vi "MT Measure QAM Quadrature Impairments.vi"(0 "recovered complex waveform":T6={"t0"=0.0, "dt"=1.0, "Y"=[]} {"Y" format="%.3f"; "dt" format="%^.2e"; "t0" format="%.4f"}, 1 "QAM system parameters":T3={"samples per symbol (16)"=16, "symbol map"=[]} {"symbol map" format="%.3f"}, 5 "input bit stream":i8[](array[numeric]), 7 "impairment measurement window":T4={"start index (symbols)"=0, "width (symbols) (-1: all)"=-1}, 9 "EVM normalization type":enum16{"Peak ", "RMS "}(ring), 11 "error in (no error)":errorcluster, 12 "impairment definition":enum16{"Vertical Shear", "Axis Shear"}(ring), 13 "reset? (T)":bool=TRUE) -> (2 "magnitude error":T1 {"individual symbol measurements (%)" format="%.2f"; "peak measurement (%)" format="%.2f"; "RMS measurement (%)" format="%.2f"}, 3 "DC offset measurements":T5 {"origin offset (dB)" format="%.2f"; "Q (%)" format="%.2f"; "I (%)" format="%.2f"}, 4 "IQ gain imbalance (dB)":dbl format="%.2f", 6 "phase error":T2 {"individual symbol measurements (deg)" format="%.2f"; "peak measurement (deg)" format="%.2f"; "RMS measurement (deg)" format="%.2f"}, 8 "EVM":T1 {"individual symbol measurements (%)" format="%.2f"; "peak measurement (%)" format="%.2f"; "RMS measurement (%)" format="%.2f"}, 10 "modulation error ratio (dB)":dbl format="%.2f", 14 "quadrature skew (deg)":dbl format="%.2f", 15 "error out":errorcluster)   [LabVIEW 2020, in "niDMT.lvlib"]
doc: "This polymorphic instance calculates and reports quadrature-amplitude modulation (QAM) quadrature impairments."
uses:
  <vilib>/addons/Modulation/niDMT.lvlib
  <vilib>/addons/Modulation/Analog/controls/Complex Data Waveform.ctl
  <vilib>/addons/Modulation/niAMT.lvlib
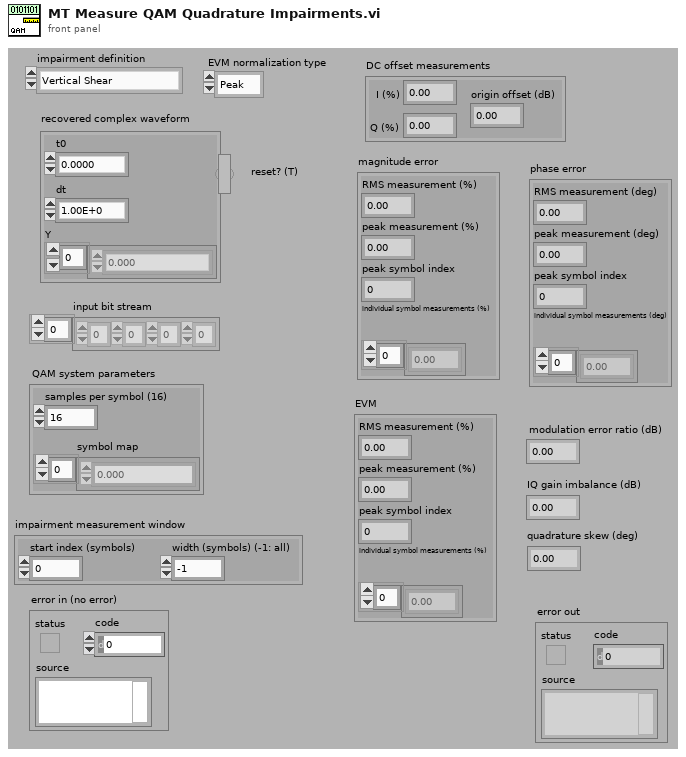
[diagram p1: front panel]
types:
  T1 = cluster{"RMS measurement (%)":dbl, "peak measurement (%)":dbl, "peak symbol index":i32, "individual symbol measurements (%)":dbl[]}
  T2 = cluster{"RMS measurement (deg)":dbl, "peak measurement (deg)":dbl, "peak symbol index":i32, "individual symbol measurements (deg)":dbl[]}
  T3 = cluster{"samples per symbol (16)":i32, "symbol map":cdb[]}
  T4 = cluster{"start index (symbols)":i32, "width (symbols) (-1: all)":i32}
  T5 = cluster{"I (%)":dbl, "Q (%)":dbl, "origin offset (dB)":dbl}
  T6 = typedef "niAMT.lvlib/Complex Data Waveform.ctl" = cluster{"t0":dbl, "dt":dbl, "Y":cdb[]}
  T7 = enum16{"FSK", "PSK", "QAM", "MSK", "PAM", "ASK", "CPM"}
  T8 = cluster{"I, %":dbl, "Q, %":dbl, "Origin Offset, dB":dbl}
  T9 = cluster{"RMS Measurement, %":dbl, "Peak Measurement, %":dbl, "Peak Symbol Index":i32, "Individual Symbol Measurements, %":dbl[]}
  T10 = cluster{"RMS Measurement, deg":dbl, "Peak Measurement, deg":dbl, "Peak Symbol Index":i32, "Individual Symbol Measurements, deg":dbl[]}
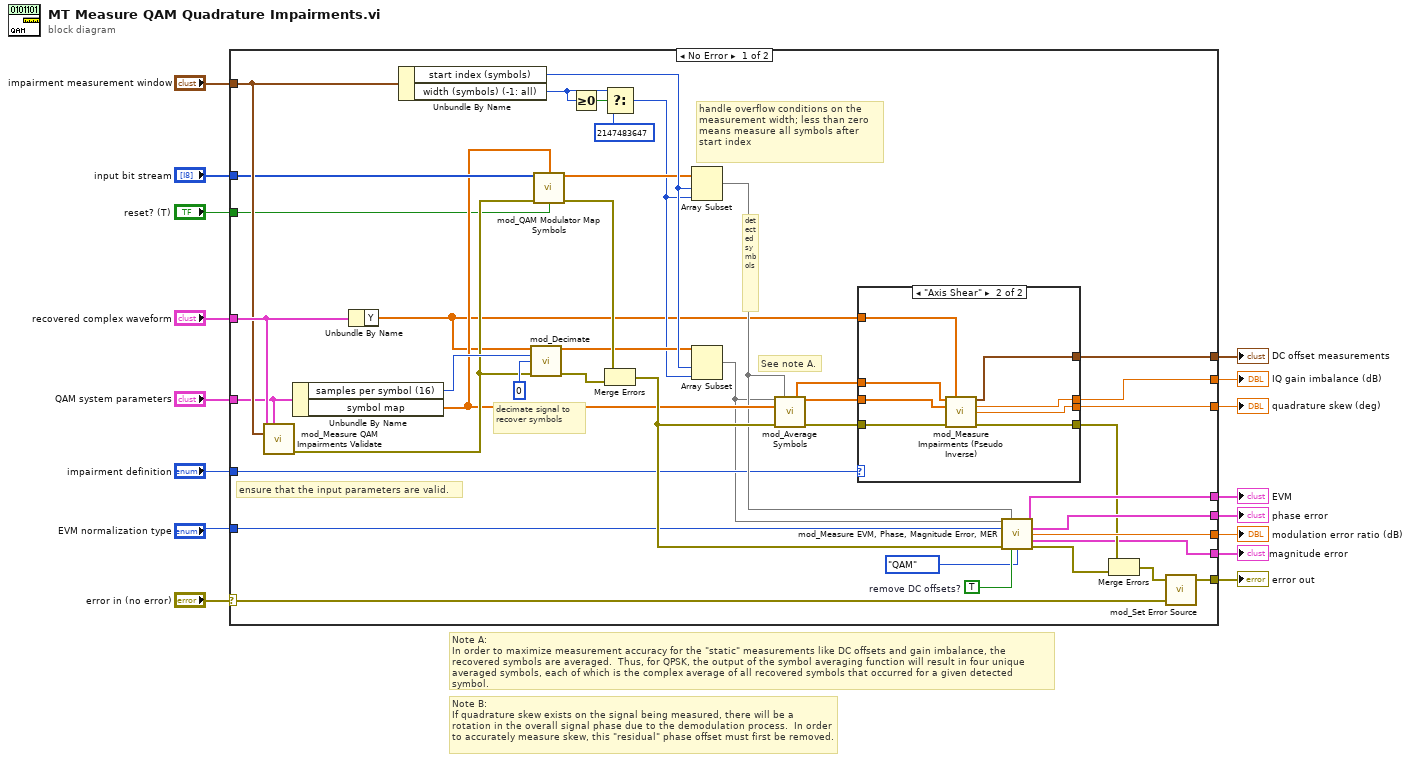
[diagram p0: block diagram]
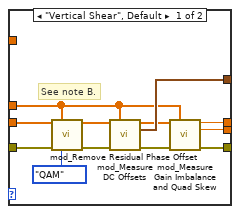
[diagram p2: hidden frame]
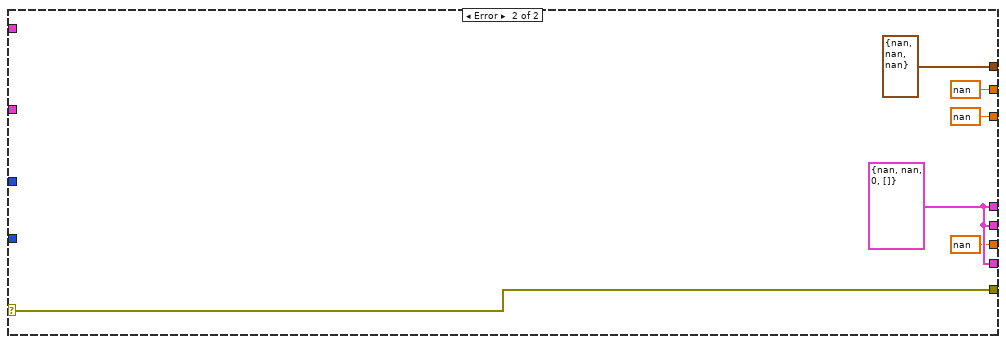
[diagram p3: hidden frame]
diagram:
  # "Note B:\nIf quadrature skew exists on the signal being measured, there will be a rotation in the overall signal phase due to the demodulation process.  In order to accurately measure skew, this \"residual\" phase offset must first be removed."
  # "Note A:\nIn order to maximize measurement accuracy for the \"static\" measurements like DC offsets and gain imbalance, the recovered symbols are averaged.  Thus, for QPSK, the output of the symbol averaging function will result in four unique averaged symbols, each of which is the complex average of all recovered symbols that occurred for a given detected symbol."
  n1 = case shown="No Error" "error in (no error)" {
    selector: "error in (no error)" -> [w48 w83]
    tunnel: "recovered complex waveform" -> [w55 _]
    tunnel: [w50 T8 {"I, %"=nan, "Q, %"=nan, "Origin Offset, dB"=nan} ("DC Offset Measurements")] -> w10
    tunnel: [w52 w79] -> w8
    tunnel: [w57 w79] -> w9
    tunnel: [w44 nan ("IQ gain imbalance (dB)")] -> w7
    tunnel: [w47 w83] -> w15
    tunnel: "input bit stream" -> [w40 _]
    tunnel: "impairment measurement window" -> [w53 _]
    tunnel: [w51 nan ("Modulation Error Ratio, dB")] -> w5
    tunnel: [w45 nan ("quadrature skew (deg)")] -> w6
    tunnel: "QAM system parameters" -> [w43 _]
    tunnel: "reset? (T)" -> [w27 _]
    tunnel: [w22 w79] -> w3
    tunnel: "impairment definition" -> [w21 _]
    tunnel: "EVM normalization type" -> [w17 _]
    frame No Error {
      w28 = TRUE  # remove DC offsets?
      # "decimate signal to recover symbols"
      # "See note A."
      # "ensure that the input parameters are valid."
      # "detected symbols"
      # "handle overflow conditions on the\nmeasurement width; less than zero\nmeans measure all symbols after\nstart index"
      n2 = call <vilib>:"mod_Measure QAM Impairments Validate.vi"("Input Complex Waveform"=w55, "QAM System Parameters"=w43, "Impairment Measurement Window"=w53) -> ("error out"=w38:errorcluster)  [unwired: 12 out]
      n3 = Unbundle By Name(w43) -> ("samples per symbol (16)"=w42:i32, "symbol map"=w30:cdb[])
      n4 = Unbundle By Name(w55) -> ("Y"=w18:cdb[])
      n5 = Unbundle By Name(w53) -> ("start index (symbols)"=w54:i32, "width (symbols) (-1: all)"=w23:i32)
      n6 = call <vilib>:"mod_Decimate.vi"("Signal In"=w18, "Samples Per Symbol (16)"=w42, "Offset"=0, "error in (no error)"=w38) -> ("Signal Out"=w35:cdb[], "error out"=w34:errorcluster)  [unwired: 1 in, 9 out]
      n7 = call <vilib>:"mod_QAM Modulator Map Symbols.vi"("Input Bit Stream"=w40, "Symbol Map"=w30, "error in (no error)"=w38, "Reset? (T)"=w27) -> ("Symbols"=w39:cdb[], "error out"=w37:errorcluster)  [unwired: 1 in, 9 out]
      n8 = Greater Or Equal To 0?(x=w23) -> (x >= 0?=w26:bool)
      n9 = Select(t=w23, s=w26, f=2147483647) -> (s? t:f=w24:i32)
      n10 = Merge Errors(w37, w34) -> (w36:errorcluster)
      n11 = Array Subset(array=w39, index=w54, length=w24) -> (w29:cdb[])
      n12 = Array Subset(array=w35, index=w54, length=w24) -> (w19:cdb[])
      n13 = call <vilib>:"mod_Average Symbols.vi"("Recovered Symbols"=w19, "Detected Symbols"=w29, "Symbol Map"=w30, "error in (no error)"=w36) -> ("Grouped Detected Symbols"=w32:cdb[], "Averaged Symbols"=w31:cdb[], "error out"=w33:errorcluster)  [unwired: 9 out]
      n14 = case shown="\"Axis Shear\"" w21 {
        tunnel: [w68 w73] -> w50
        tunnel: [w67 w74] -> w46
        tunnel: [w66 w71] -> w45
        tunnel: [w65 w72] -> w44
        tunnel: w33 -> [w64 w75]
        tunnel: w32 -> [w62 w77]
        tunnel: w31 -> [w61 w76]
        tunnel: w18 -> [_ w70]
        frame "Vertical Shear", Default {
          # "See note B."
          n15 = call <vilib>:"mod_Remove Residual Phase Offset.vi"("Averaged Symbols In"=w61, "Grouped Detected Symbols"=w62, "error in (no error)"=w64, "Modulation Type"=T7."QAM") -> ("Averaged Symbols Out"=w60:cdb[], "error out"=w63:errorcluster)  [unwired: 10 out]
          n16 = call <vilib>:"mod_Measure DC Offsets.vi"("Averaged Symbols"=w60, "Grouped Detected Symbols"=w62, "error in (no error)"=w63) -> ("Corrected Symbols"=w59:cdb[], "DC Offset Measurements"=w68:T8, "error out"=w69:errorcluster)  [unwired: 1 in, 9 out]
          n17 = call <vilib>:"mod_Measure Gain Imbalance and Quad Skew.vi"("Corrected Symbols"=w59, "Grouped Detected Symbols"=w62, "error in (no error)"=w69) -> ("IQ Gain Imbalance, dB"=w65:dbl, "Quadrature Skew, deg"=w66:dbl, "error out"=w67:errorcluster)  [unwired: 1 in, 9 out]
        }
        frame "Axis Shear" {
          n18 = call <vilib>:"mod_Measure Impairments (Pseudo Inverse).vi"("Grouped detected symbols"=w77, "Recovered Complex Waveform"=w70, "Averaged symbols"=w76, "error in (no error)"=w75) -> ("DC Offset Measurements"=w73:T8, "IQ gain imbalance (dB)"=w72:dbl, "quadrature skew (deg)"=w71:dbl, "error out"=w74:errorcluster)  [unwired: 1 in, 7 out]
        }
      }
      n19 = call <vilib>:"mod_Measure EVM, Phase, Magnitude Error, MER.vi"("Recovered Signal"=w19, "Detected Signal"=w29, "EVM Normalization Type"=w17, "error in (no error)"=w36, "remove DC offsets? (T)"=w28, "Modulation Type"=T7."QAM") -> ("EVM"=w57:T9, "Phase Error"=w52:T10, "Modulation Error Ratio, dB"=w51:dbl, "magnitude error"=w22:T9, "error out"=w56:errorcluster)  [unwired: 5 out]
      n20 = Merge Errors(w46, w56) -> (w49:errorcluster)
      n21 = call <vilib>:"mod_Set Error Source.vi"("initial error in (no error)"=w48, "final error in (no error)"=w49) -> ("error out"=w47:errorcluster)  [unwired: 3 out]
    }
    frame Error {
      w79 = T9 {"RMS Measurement, %"=nan, "Peak Measurement, %"=nan, "Peak Symbol Index"=0, "Individual Symbol Measurements, %"=[]} ("EVM")
    }
  }
  "error out" <- w15
  "IQ gain imbalance (dB)" <- w7
  "quadrature skew (deg)" <- w6
  "modulation error ratio (dB)" <- w5
  "DC offset measurements" <- w10
  "EVM" <- w9
  "phase error" <- w8
  "magnitude error" <- w3
